vi "lib Fix End-of-Line.vi"(11 "File":path) -> (2 "number of replacements":i32, 3 "File dup":path)   [LabVIEW 2011]
panel:
  out "text":string
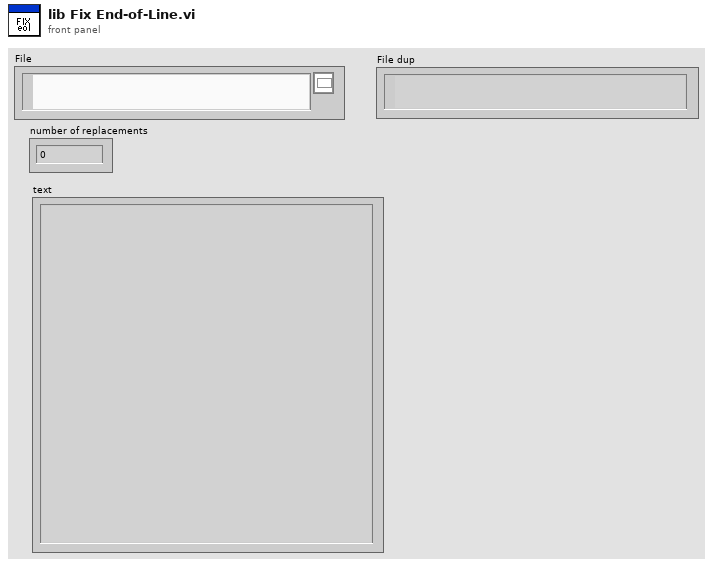
[diagram p1: front panel]
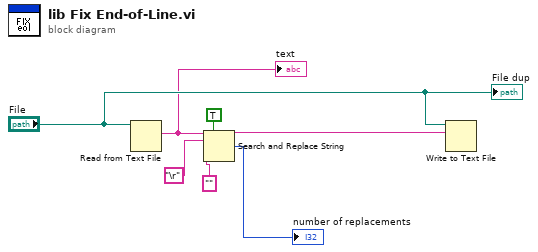
[diagram p0: block diagram]
diagram:
  n1 = Read from Text File(file (use dialog)="File") -> (text=w1:string)  [unwired: 3 in, 3 out]
  "text" <- w1
  n2 = Search and Replace String(replace all?=TRUE ("replace all? (F)"), input string=w1, search string="\r", replace string="" ("replace string (\"\")")) -> (result string=w5:string, number of replacements=→"number of replacements":i32)  [unwired: 4 in, 2 out]
  n3 = Write to Text File(file (use dialog)="File", text=w5) -> ()  [unwired: 2 in, 3 out]
  "File dup" <- "File"
